vi "LinxGetDeviceName.vi"(8 "Error In":errorcluster, 11 "LINX Resource":T1) -> (0 "Error Out":errorcluster, 2 "Device Name":string, 3 "LINX Resource":T1)   [LabVIEW 2014, in "LMH-LINX.lvlib" / "Local IO.lvlib"]
uses:
  Local IO.lvlib
  Type Defs/LINX Ref.ctl
  Type Defs/Platform.ctl
  Type Defs/Interface.ctl
  Device/Type Defs/LINX Device Config.ctl
  Device/Type Defs/TCP Config.ctl
  Device/Type Defs/Channels.ctl
  Type Defs/Error Type.ctl
  liblinxdevice.dll
  LMH-LINX.lvlib
  Device/Device.lvlib
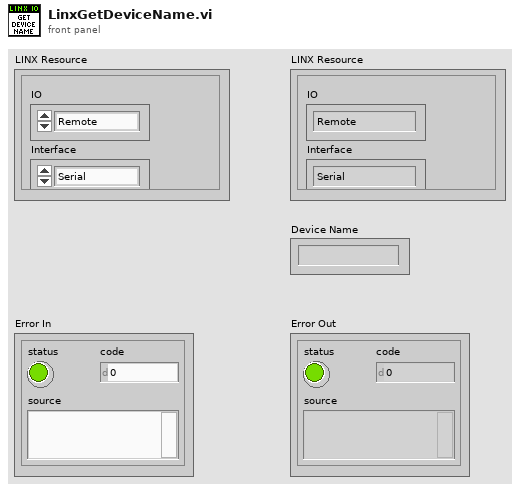
[diagram p1: front panel]
types:
  T1 = typedef "LMH-LINX.lvlib/LINX Ref.ctl" = cluster{"IO":T2, "Interface":T3, "LINX Device Config":T4}
  T2 = typedef "LMH-LINX.lvlib/Platform.ctl" = enum16{"Remote", "Local"}
  T3 = typedef "LMH-LINX.lvlib/Interface.ctl" = enum16{"Serial", "TCP"}
  T4 = typedef "LMH-LINX.lvlib/Device.lvlib/LINX Device Config.ctl" = cluster{"Interface":T3, "COM Port":refnum<visa-resource-name>, "TCP Configuration":T5, "Device Family":u8, "Device ID":u8, "Device Name":string, "TCP Ref":refnum<k5>, "Channels":T6}
  T5 = typedef "LMH-LINX.lvlib/Device.lvlib/TCP Config.ctl" = cluster{"IP Address":string, "Port":u16}
  T6 = typedef "LMH-LINX.lvlib/Channels.ctl" = cluster{"DI":u8[], "DO":u8[], "AI":u8[], "AO":u8[], "PWM":u8[], "QE":u8[], "UART":u8[], "I2C 2":u8[], "SPI":u8[], "CAN":u8[], "Servo":u8[], "AI Ref (V)":dbl, "AI Resolution (Bits)":u8, "AO Ref (V)":dbl, "AO Resolution (Bits)":u8}
  T7 = typedef "LMH-LINX.lvlib/Error Type.ctl" = enum16{"Unknown", "Timeout", "Corrupt Return Packet", "Unable To Connect", "Command Not Supported", "Channel DNE", "Invalid COM Config", "Firmware Version Mismatch", "myRIO Support", "CMD Specific Error", "Local IO Not Supported"}
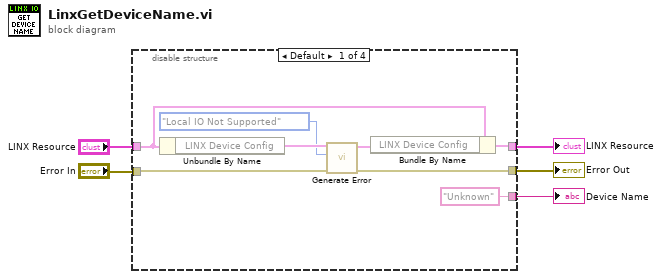
[diagram p0: block diagram]
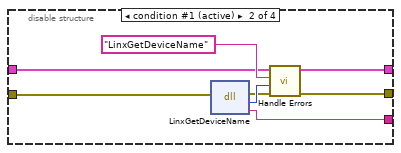
[diagram p2: hidden frame]
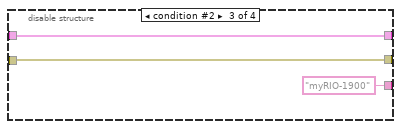
[diagram p3: hidden frame]
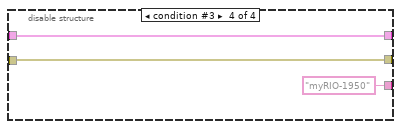
[diagram p4: hidden frame]
diagram:
  n1 = disable-structure shown="Default" {
    disable-tunnel: [w11 w18 w22 w25] -> w5
    disable-tunnel: ["Unknown" ("Device Name") w17 "myRIO-1900" ("Device Name") "myRIO-1950" ("Device Name")] -> w4
    disable-tunnel: [w8 w16 w23 w26] -> w3
    disable-tunnel: "LINX Resource" -> [w12 w15 w22 w25]
    disable-tunnel: "Error In" -> [w9 w14 w23 w26]
    frame condition #0 {
      n2 = Unbundle By Name(w12) -> ("LINX Device Config"=w10:T4)
      n3 = call "Generate Error.vi"("Error In"=w9, "Error Type"=Error_Type."Local IO Not Supported", "LINX Device Config"=w10) -> ("Error Out"=w8:errorcluster, "Dup LINX Device Config"=w13:T4)  [unwired: 7 in]
      n4 = Bundle By Name(cluster=w12, "LINX Device Config"=w13) -> (w11:T1)
    }
    frame condition #1 (active) {
      n5 = dll-call lib="liblinxdevice.*" fn="LinxGetDeviceName"(error in=w14) -> (error out=w19:errorcluster, "LinxStatus"=w20:i32, "name"=w17:string)  [unwired: 3 in, 1 out]
      n6 = call "Handle Errors.vi"("Error In"=w19, "LinxStatus"=w20, "Function Name"="LinxGetDeviceName", "LINX Resource"=w15) -> ("Error Out"=w16:errorcluster, "LINX Resource"=w18:T1)  [unwired: 6 in]
    }
    frame condition #2 {
    }
    frame condition #3 {
    }
  }
  "Error Out" <- w3
  "LINX Resource" <- w5
  "Device Name" <- w4
